vi "Registration Info from Disk.vi"(0 "reference in":refnum<class "Registration.lvclass">, 5 "error in (no error)":errorcluster) -> (13 "Registration Info":T1, 14 "reference OUT":refnum<class "Registration.lvclass">, 19 "error out":errorcluster)   [LabVIEW 2022 SP3, in "Registration.lvclass"]
uses:
  Registration.lvclass
  protected/Registration Info.ctl
  Registration Type.ctl
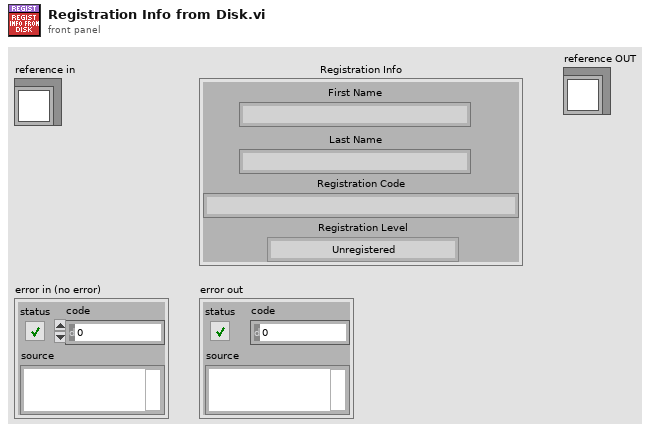
[diagram p1: front panel]
types:
  T1 = typedef "Registration.lvclass/Registration Info.ctl" = cluster{"First Name":string, "Last Name":string, "Registration Code":string, "Registration Level":T2}
  T2 = typedef "Registration.lvclass/Registration Type.ctl" = enum16{"Unregistered", "Registered - Full Activation", "Not Required- Full Activation"}
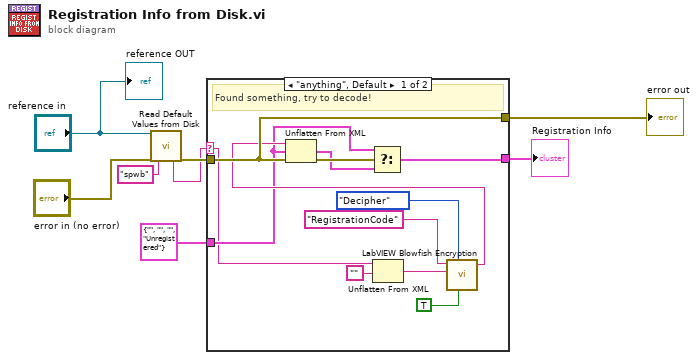
[diagram p0: block diagram]
diagram:
  n1 = call-dynamic "Read Default Values from Disk.vi"("reference in"="reference in", "error in (no error)"="error in (no error)", "Control Label"="spwb" ("Filename")) -> ("Value (XML String)"=w1:string, "error out"=w3:errorcluster)  [unwired: 14 in, 1 out]
  n2 = case shown="\"anything\", Default" w1 {
    selector: w1 -> [w11 _]
    tunnel: w3 -> [w19 w22]
    tunnel: [w19 w22] -> w8
    tunnel: T1 {"First Name"="", "Last Name"="", "Registration Code"="", "Registration Level"=enum."Unregistered"} ("Registration Info") -> [w12 w21]
    tunnel: [w13 w21] -> w6
    frame "anything", Default {
      # "Found something, try to decode!"
      n3 = Unflatten From XML(xml string=w11, type="") -> (value=w9:string)  [unwired: 1 in, 1 out]
      n4 = call "LabVIEW Blowfish Encryption.vi"("Password"="RegistrationCode", "Enc/Dec"=enum16{"Encipher", "Decipher"}."Decipher", "Input Text"=w9, "Output As ASCII\nfor email Transmission"=TRUE ("Output As ASCII\nfor email Transmission")) -> ("Output text"=w14:string)  [unwired: 2 in, 2 out]
      n5 = Unflatten From XML(xml string=w14, type=w12, error in (no error)=w19) -> (value=w18:T1, error out=w20:errorcluster)
      n6 = Select(t=w12, s=w20, f=w18) -> (s? t:f=w13:T1)
    }
    frame "" {
      # "Either the file was not found or there was some error"
    }
  }
  "error out" <- w8
  "Registration Info" <- w6
  "reference OUT" <- "reference in"
